vi "Store Static VI References for Subpanel.vi"(8 "error in (no error)":errorcluster, 11 "Motions Configuration in":refnum<class "Motions Configuration.lvclass">) -> (0 "error out":errorcluster, 3 "Motions Configuration out":refnum<class "Motions Configuration.lvclass">)   [LabVIEW 2016, in "Hardware.lvlib" / "Motions.lvlib" / "Motions Configuration.lvclass"]
uses:
  <userlib>/Common Components/Hardware/Abstract System/Motions/Motions Config/Motions Configuration.lvclass
  <userlib>/Configuration Dialog Actor/Configuration.lvclass
  C:/Program Files (x86)/National Instruments/LabVIEW 2016/user.lib/Configuration Dialog Actor/Configuration.lvclass
  C:/Program Files (x86)/National Instruments/LabVIEW 2016/vi.lib/ActorFramework/Actor/Actor.lvclass
  <userlib>/Common Components/Hardware/Motor/Motor Config/Motor Configuration.lvclass
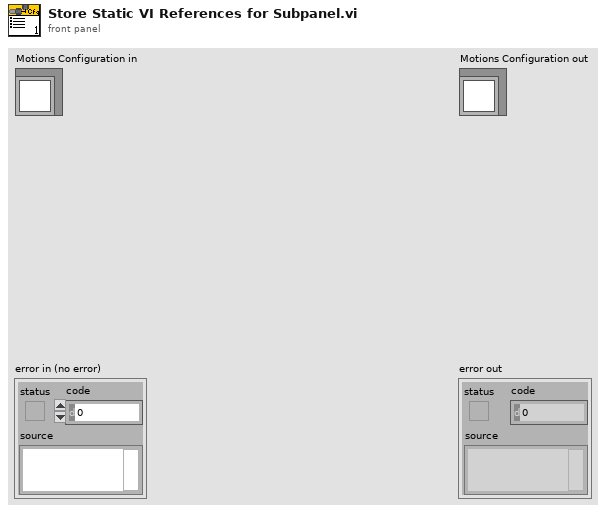
[diagram p1: front panel]
types:
  T1 = typedef "Configuration.lvlib/Configuration.lvclass/Data Retrieved by Lookup Table.ctl" = cluster{"VI Refnum":refnum<vi>, "Help Text":string}
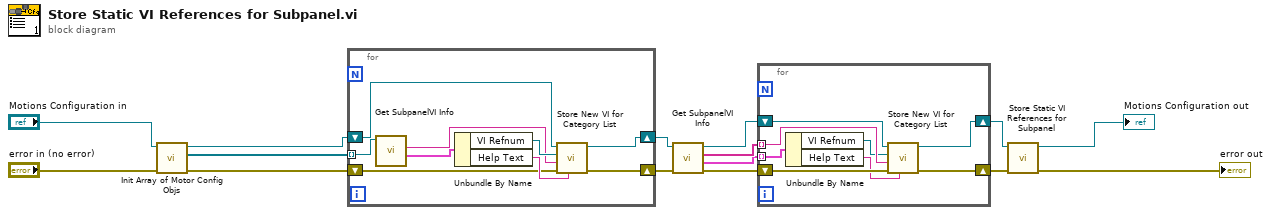
[diagram p0: block diagram]
diagram:
  n1 = call <userlib>:"Init Array of Motor Config Objs.vi"("error in (no error)"="error in (no error)", "Motions Configuration in"="Motions Configuration in") -> ("error out"=w2:errorcluster, "Array of Motor Config Objs"=w5:refnum<class "Motor Configuration.lvclass">[], "Motions Configuration out"=w4:refnum<class "Motions Configuration.lvclass">)  [unwired: 7 in]
  n2 = for {
    tunnel: w5 -> [w24] mode=indexing
    shift-right: [w19] -> w3
    shift-left: w4 -> [w20]
    shift-right: [w17] -> w1
    shift-left: w2 -> [w18]
    n3 = call-dynamic "Get SubpanelVI Info.vi"("Motor Configuration in"=w24) -> ("Subpanel VI data"=w21:T1, "Category string"=w16:string)  [unwired: 7 in, 2 out]
    n4 = Unbundle By Name(w21) -> ("VI Refnum"=w23:refnum<vi>, "Help Text"=w22:string)
    n5 = call <userlib>:"Store New VI for Category List.vi"("Help Text"=w22, "error in (no error)"=w18, "String"=w16, "VI Refnum"=w23, "Configuration in"=w20) -> ("error out"=w17:errorcluster, "Configuration out"=w19:refnum<class "Motions Configuration.lvclass">)  [unwired: 5 in]
  }
  n6 = call-dynamic "Get SubpanelVI Info.vi"("error in (no error)"=w1, "Motions Configuration in"=w3) -> ("error out"=w10:errorcluster, "Array of Subpanel VI data"=w7:T1[], "Array of Category string"=w8:string[], "Motions Configuration out"=w12:refnum<class "Motions Configuration.lvclass">)  [unwired: 6 in]
  n7 = for {
    tunnel: w7 -> [w28] mode=indexing
    shift-right: [w31] -> w9
    shift-left: w10 -> [w32]
    shift-right: [w29] -> w11
    shift-left: w12 -> [w30]
    tunnel: w8 -> [w27] mode=indexing
    n8 = Unbundle By Name(w28) -> ("VI Refnum"=w26:refnum<vi>, "Help Text"=w25:string)
    n9 = call <userlib>:"Store New VI for Category List.vi"("Help Text"=w25, "error in (no error)"=w32, "String"=w27, "VI Refnum"=w26, "Configuration in"=w30) -> ("error out"=w31:errorcluster, "Configuration out"=w29:refnum<class "Motions Configuration.lvclass">)  [unwired: 5 in]
  }
  n10 = call-parent "Store Static VI References for Subpanel.vi"("error in (no error)"=w9, "Configuration in"=w11) -> ("error out"=→"error out":errorcluster, "Configuration out"=→"Motions Configuration out":refnum<class "Motions Configuration.lvclass">)  [unwired: 8 in]
